vi "qar wave gen.vi"() -> ()   [LabVIEW 2019]
uses:
  <vilib>/measure/NI_MABase.lvlib
panel:
  out "Waveform Graph 2":waveform(dbl)(graph)
  out "x+y 2":waveform(dbl)
  out "signal out":waveform(dbl)
  out "x+y":waveform(dbl)
  out "Waveform Graph":waveform(dbl)(graph)
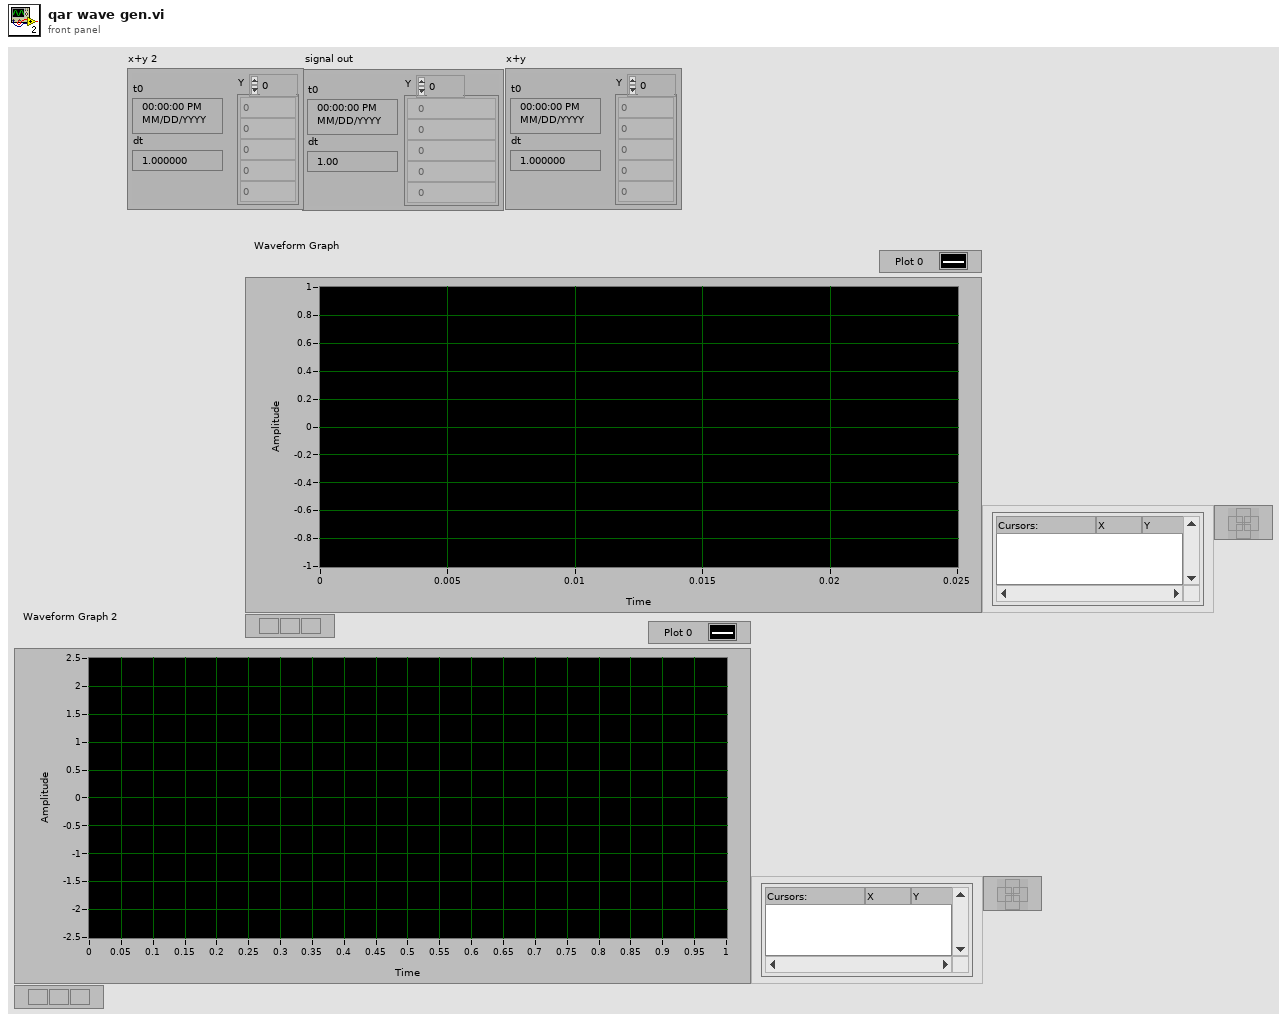
[diagram p1: front panel]
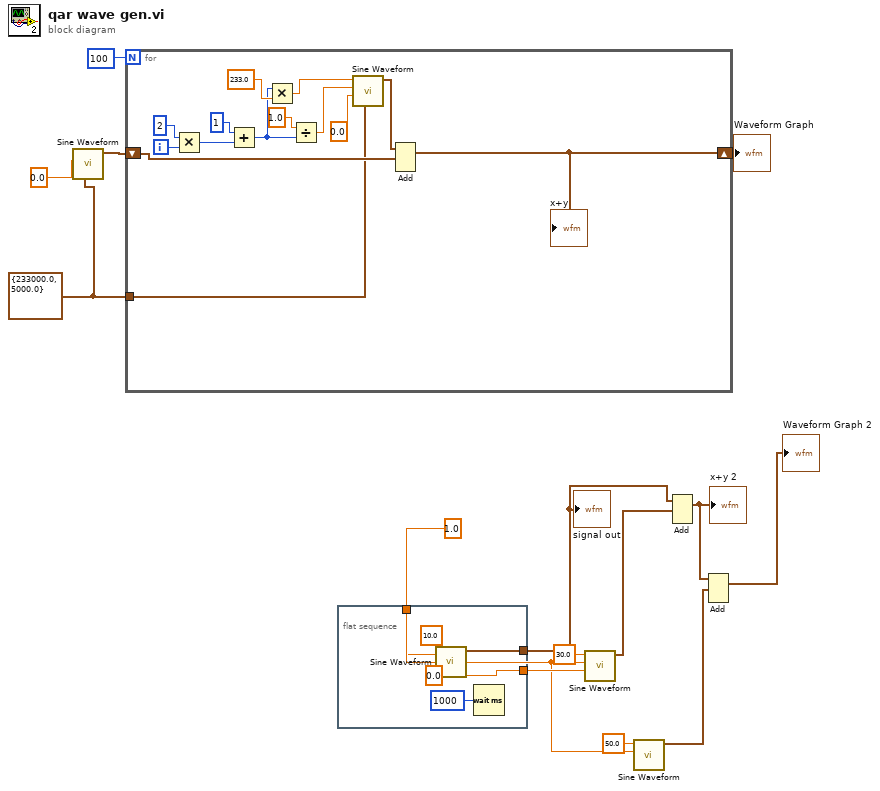
[diagram p0: block diagram]
diagram:
  w1 = cluster{"Fs":dbl, "#s":dbl} {"Fs"=233000.0, "#s"=5000.0} ("sampling info")
  w4 = 1.0 ("amplitude")
  n1 = call <vilib>:"Sine Waveform.vi"("sampling info"=w1, "amplitude"=0.0) -> ("signal out"=w12:waveform(dbl))  [unwired: 8 in, 1 out]
  n2 = for {
    N: 100 -> [_]
    shift-right: [w17] -> w11
    shift-left: w12 -> [w18]
    tunnel: w1 -> [w15]
    i -> [w22]
    n3 = Multiply(x=2, y=w22) -> (x*y=w21:i32)
    n4 = Add(x=1, y=w21) -> (x+y=w20:i32)
    n5 = Multiply(x=w20, y=233.0 ("frequency")) -> (x*y=w16:dbl)
    n6 = Divide(x=1.0 ("amplitude"), y=w20) -> (x/y=w23:dbl)
    n7 = call <vilib>:"Sine Waveform.vi"("sampling info"=w15, "phase"=0.0, "amplitude"=w23, "frequency"=w16) -> ("signal out"=w19:waveform(dbl))  [unwired: 6 in, 1 out]
    n8 = Add(1:w18, 2:w19) -> (0:w17:waveform(dbl))  [unwired: 1 in, 1 out]
    "x+y" <- w17
  }
  "Waveform Graph" <- w11
  n9 = flat-sequence {
    tunnel: w4 -> [w33]
    tunnel: [w32] -> w10
    tunnel: [w31] -> w8
    frame #0 {
      w32 = 0.0 ("phase")
      n10 = call <vilib>:"Sine Waveform.vi"("phase"=w32, "amplitude"=w33, "frequency"=10.0) -> ("signal out"=w31:waveform(dbl))  [unwired: 7 in, 1 out]
      n11 = Wait (ms)(milliseconds to wait=u32 1000) -> ()  [unwired: 1 out]
    }
  }
  n12 = call <vilib>:"Sine Waveform.vi"("phase"=w10, "amplitude"=w4, "frequency"=30.0) -> ("signal out"=w9:waveform(dbl))  [unwired: 7 in, 1 out]
  n13 = call <vilib>:"Sine Waveform.vi"("amplitude"=w4, "frequency"=50.0) -> ("signal out"=w5:waveform(dbl))  [unwired: 8 in, 1 out]
  n14 = Add(1:w9, 2:w8) -> (0:w6:waveform(dbl))  [unwired: 1 in, 1 out]
  "x+y 2" <- w6
  n15 = Add(1:w5, 2:w6) -> (0:→"Waveform Graph 2":waveform(dbl))  [unwired: 1 in, 1 out]
  "signal out" <- w8
